vi "Read Card ID.vi"(0 "COM":refnum<visa-resource-name>, 1 "Timeout (ms)":u32=500, 7 "Address":string="01", 11 "error in (no error)":errorcluster) -> (4 "COM OUT":refnum<visa-resource-name>, 6 "ReceiveString":string, 15 "error out":errorcluster)   [LabVIEW 2020, in "Reader.lvlib"]
uses:
  Reader.lvlib
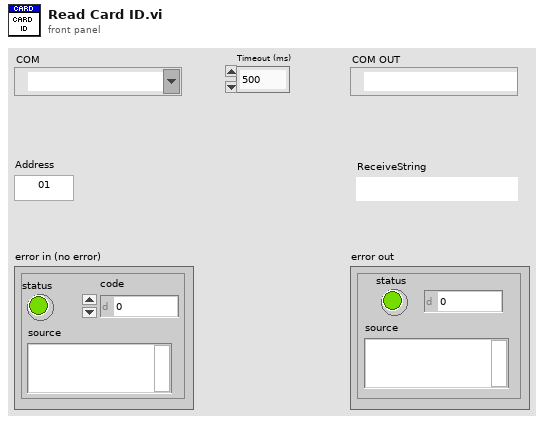
[diagram p1: front panel]
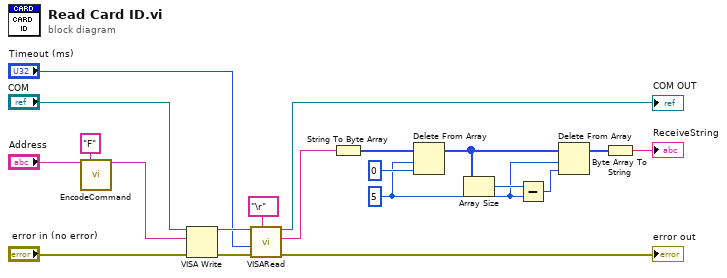
[diagram p0: block diagram]
diagram:
  w3 = 5 ("length (len. of substring)")
  n1 = call "EncodeCommand.vi"("Address"="Address", "Function"="F") -> ("Command String"=w15:string)  [unwired: 12 in, 1 out]
  n2 = VISA Write(VISA resource name="COM", write buffer=w15, error in (no error)="error in (no error)") -> (VISA resource name out=w17:refnum<visa-resource-name>, error out=w16:errorcluster)  [unwired: 1 out]
  n3 = call "VISARead.vi"("Termination Char (blank)"="\r" ("Read regular"), "error in (no error)"=w16, "Timeout (ms)"="Timeout (ms)", "Resource in"=w17) -> ("error out"=→"error out":errorcluster, "Read Char"=w9:string, "Resource out"=→"COM OUT":refnum<visa-resource-name>)  [unwired: 5 in]
  n4 = String To Byte Array(string=w9) -> (unsigned byte array=w8:u8[])
  n5 = Delete From Array(array=w8, length=w3, index=0) -> (array with subset deleted=w5:u8[])  [unwired: 1 out]
  n6 = Array Size(array=w5) -> (size(s)=w4:i32)
  n7 = Subtract(x=w4, y=w3) -> (x-y=w2:i32)
  n8 = Delete From Array(array=w5, length=w3, index=w2) -> (array with subset deleted=w1:u8[])  [unwired: 1 out]
  n9 = Byte Array To String(unsigned byte array=w1) -> (string=→"ReceiveString":string)
